vi "MMEM_STOR_TRAC_FORM_SNP.vi"(0 "VISA IN":refnum<visa-resource-name>, 5 "error in":errorcluster, 7 "Format":string(combo)="AUTO") -> (14 "VISA Out":refnum<visa-resource-name>, 19 "error out":errorcluster)   [LabVIEW 2018, in "PNA-X.lvlib"]
doc: "MMEMory:STORe:TRACe:FORMat:SNP <char> \n(Read-Write) Specifies the format of subsequent .s1p, .s2p, .s3p; s4p save statements. (See Data \nDefine Saves). \nParameters \n<char> Choose from: \nMA - Linear Magnitude / degrees \nDB - Log Magnitude / degrees \nRI - Real / Imaginary \nAUTO - data is output in currently selected trace format. If other than LogMag, \nLinMag, or Real/Imag, then output is in Real/Imag. \nExamples MMEM:STOR:TRAC:FORM:SNP MA \nQuery Syntax MMEMory:STORe:TRACe:FORMat:SNP? \nReturn Type Character \nDefault Auto' \n1615"
uses:
  PNA-X.lvlib
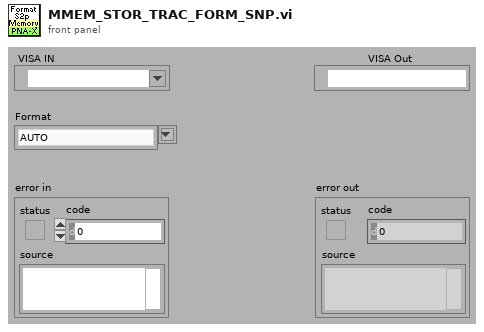
[diagram p1: front panel]
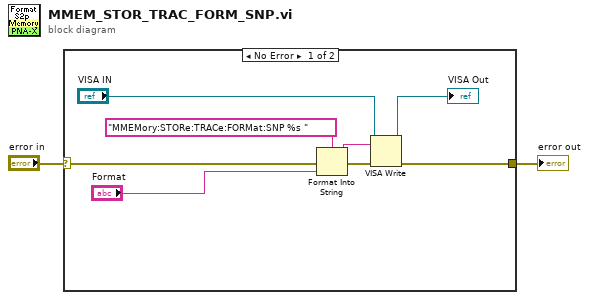
[diagram p0: block diagram]
diagram:
  n1 = case shown="No Error" "error in" {
    selector: "error in" -> [w10 w11]
    tunnel: [w5 w11] -> w1
    frame No Error {
      n2 = Format Into String(format string="MMEMory:STORe:TRACe:FORMat:SNP %s " ("Cmdline"), error in=w10, "Format") -> (resulting string=w8:string, error out=w9:errorcluster)  [unwired: 1 in]
      n3 = VISA Write(VISA resource name="VISA IN", write buffer=w8, error in (no error)=w9) -> (VISA resource name out=→"VISA Out":refnum<visa-resource-name>, error out=w5:errorcluster)  [unwired: 1 out]
    }
    frame Error {
    }
  }
  "error out" <- w1
